vi "Read from Property Bag.vi"(8 "error in (no error)":errorcluster, 9 "Data in":variant, 11 "Jenkins Builder in":refnum<class "Jenkins Builder.lvclass">) -> (0 "error out":errorcluster, 3 "Jenkins Builder out":refnum<class "Jenkins Builder.lvclass">)   [LabVIEW 2014, in "Jenkins Builder.lvclass"]
uses:
  Jenkins Builder.lvclass
  CI Serializer/CI Serializer.lvclass/CI Serializer.ctl
  Jenkins Builder.lvclass/Jenkins Builder.ctl
  CI Serializer/CI Serializer.lvclass
  Shared/Classes/Status Events/Status Events.lvclass
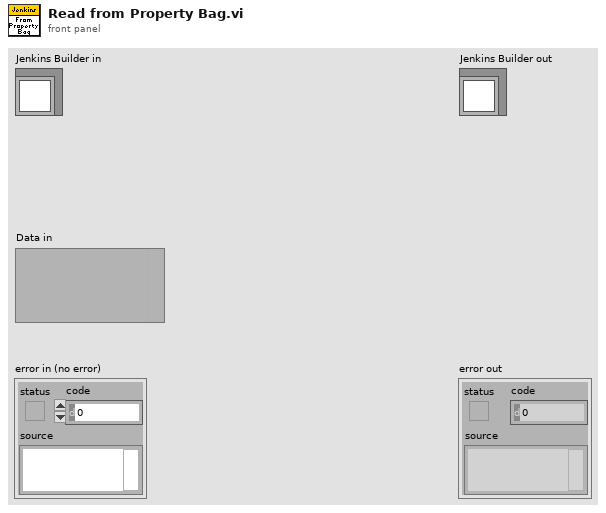
[diagram p1: front panel]
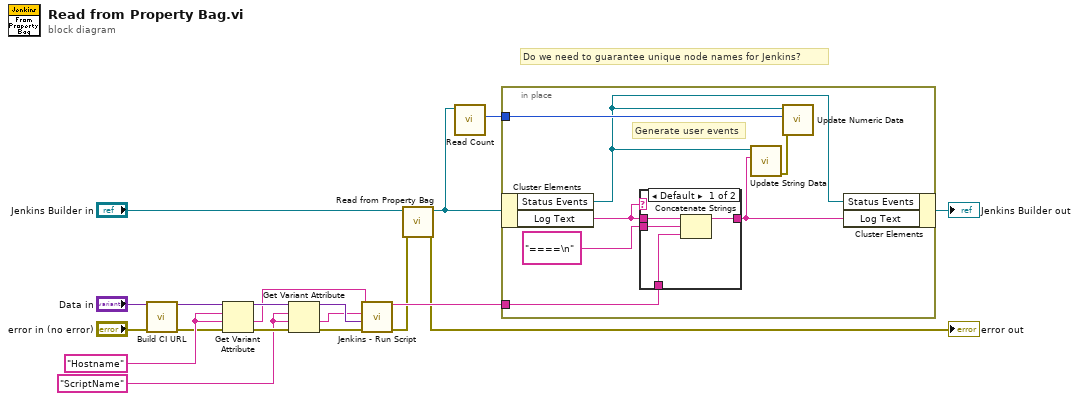
[diagram p0: block diagram]
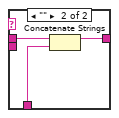
[diagram p2: hidden frame]
diagram:
  w16 = "ScriptName" ("name")
  w17 = "Hostname" ("name")
  # "Do we need to guarantee unique node names for Jenkins?"
  n1 = call "Build CI URL.vi"("error in"="error in (no error)", "Parameters"="Data in") -> ("error out"=w8:errorcluster, "Parameters out"=w6:variant)  [unwired: 8 in]
  n2 = Get Variant Attribute(Variant=w6, name=w17, default value (empty Variant)=w17, error in=w8) -> (duplicate Variant=w18:variant, value=w13:string, error out=w19:errorcluster)  [unwired: 1 out]
  n3 = Get Variant Attribute(Variant=w18, name=w16, default value (empty Variant)=w16, error in=w19) -> (duplicate Variant=w14:variant, value=w12:string, error out=w15:errorcluster)  [unwired: 1 out]
  n4 = call "Jenkins - Run Script.vi"("error in (no error)"=w15, "Parameters"=w14, "Script Job Name (Within Build Script Folder)"=w12, "IP Address"=w13) -> ("error out"=w5:errorcluster, "Text"=w10:string)  [unwired: 6 in]
  n5 = call-parent "Read from Property Bag.vi"("error in (no error)"=w5, "CI Serializer in"="Jenkins Builder in") -> ("error out"=→"error out":errorcluster, "CI Serializer out"=w1:refnum<class "Jenkins Builder.lvclass">)  [unwired: 8 in]
  n6 = call "Read Count.vi"("CI Serializer in"=w1) -> ("Count"=w3:i32)  [unwired: 10 in]
  n7 = in-place {
    in-place-border: w10 -> [w26]
    in-place-border: w3 -> [w24]
    # "Generate user events"
    n8 = in-place-cluster #1(w1) -> ("Status Events"=w23:refnum<class "Status Events.lvclass">, "Log Text"=w25:string)
    n9 = case shown="Default" w25 {
      tunnel: "====\n" ("string") -> [w30 _]
      tunnel: w25 -> [w29 w33]
      tunnel: w26 -> [w28 w32]
      tunnel: [w27 w31] -> w21
      frame Default {
        n10 = Concatenate Strings(w29, w30, w28) -> (w27:string)
      }
      frame "" {
        n11 = Concatenate Strings(w33, w32) -> (w31:string)
      }
    }
    n12 = call "Update String Data.vi"("String Data"=w21, "Status Updater in"=w23) -> ("error out"=w20:errorcluster)  [unwired: 8 in, 1 out]
    n13 = call "Update Numeric Data.vi"("error in (no error)"=w20, "Numeric Data"=w24, "Status Updater in"=w23) -> ()  [unwired: 7 in, 2 out]
    n14 = in-place-cluster #1("Status Events"=w23, "Log Text"=w21) -> (→"Jenkins Builder out":refnum<class "Jenkins Builder.lvclass">)
  }
